vi "ZK仪器状态.vi"(7 "运行模式":string, 8 "error in (no error)":errorcluster, 11 "Slave ID":T3) -> (0 "error out":errorcluster, 2 "质控仪器状态显示":T1, 3 "质控仪器状态":T2 {"当前步骤数" format="0x%04xH"})   [LabVIEW 2016, in "质控单元V4.lvlib"]
uses:
  <vilib>/Plasmionique/MB Master/MB_Master/MB_Master.lvclass
  <vilib>/Plasmionique/MB Master/MB Master.lvlib
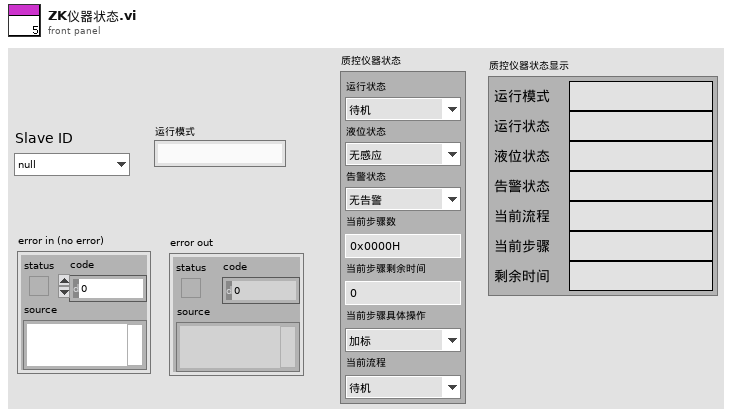
[diagram p1: front panel]
types:
  T1 = typedef "质控单元V4.lvlib/质控仪器状态显示.ctl" = cluster{"运行模式":string, "运行状态":string, "液位状态":string, "告警状态":string, "当前流程":string, "当前步骤":string, "剩余时间":string}
  T2 = typedef "质控单元V4.lvlib/质控仪器状态.ctl" = cluster{"运行状态":enum16{"待机", "润洗", "进样", "定量", "加标", "等待取样", "排液", "异常停机"}, "液位状态":enum16{"无感应", "有感应"}, "告警状态":enum16{"无告警", "液位故障告警", "注射泵异常"}, "当前步骤数":u16, "当前步骤剩余时间":u16, "当前步骤具体操作":enum16{"加标", "进样", "排液", "搅拌", "定量"}, "当前流程":enum16{"待机", "进样流程", "加标流程", "排液流程", "水样润洗流程", "加标润洗流程"}}
  T3 = typedef "质控单元V4.lvlib/质控slave id.ctl" = enum16{"null", "氨氮", "总磷", "总氮", "CODMn", "CODCr"}
  T4 = cluster{"[0]":u16, "[1]":u16, "[2]":u16, "[3]":u16, "[4]":u16, "[5]":u16, "[6]":u16}
  T5 = enum16{"待机", "润洗", "进样", "定量", "加标", "等待取样", "排液", "异常停机"}
  T6 = cluster{"运行模式":string, "RingText.Text":string, "RingText.Text":string, "RingText.Text":string, string, "RingText.Text":string, string}
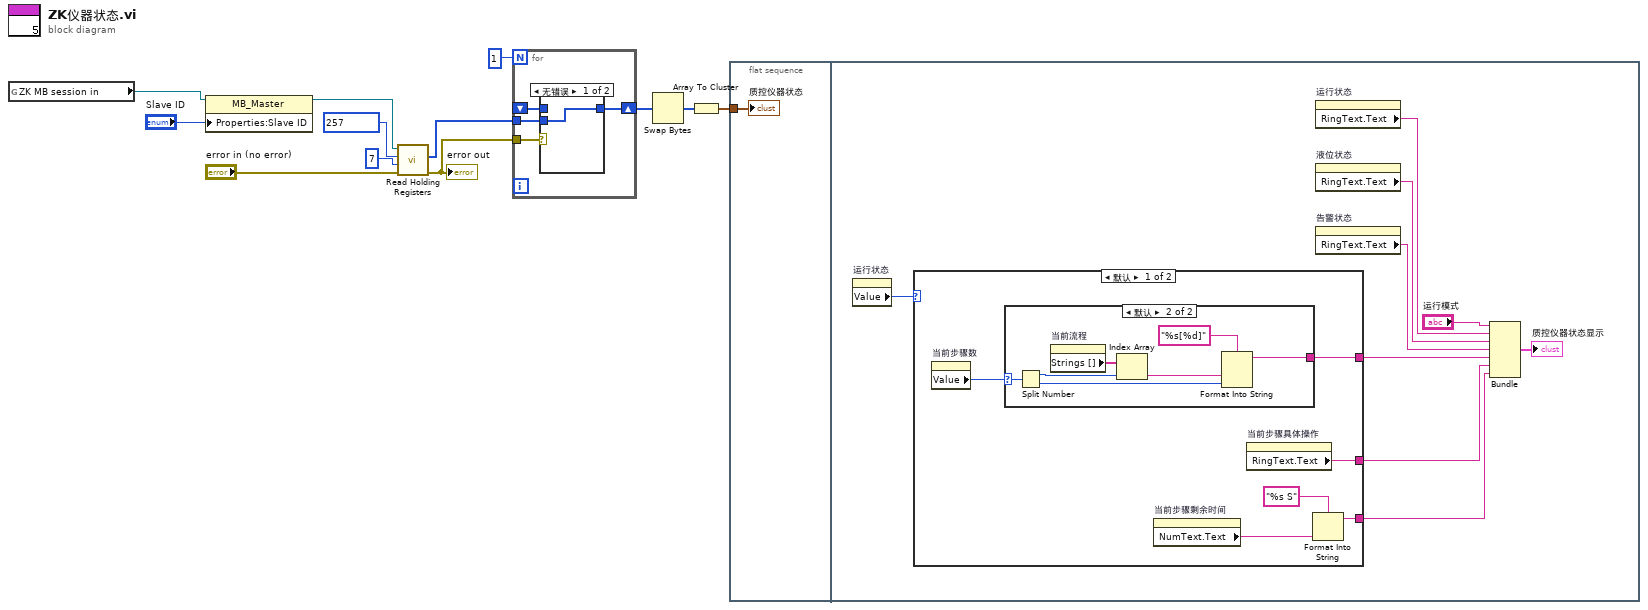
[diagram p0: block diagram]
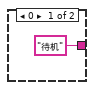
[diagram p2: hidden frame]
diagram:
  n1 = global read "ZK非断电保存全局变量.vi" "ZK MB session in"() -> (w11:refnum<class "MB_Master.lvclass">)
  n2 = property class="MB_Master"(reference=w11, "Properties:Slave ID"="Slave ID") -> (reference out=w9:refnum<class "MB_Master.lvclass">)  [unwired: 1 in, 1 out]
  n3 = call <vilib>:"Read Holding Registers.vi"("error in (no error)"="error in (no error)", "quantity"=u16 7, "starting address"=u16 257, "MB session in"=w9) -> ("error out"=w6:errorcluster, "Registers"=w5:u16[])  [unwired: 5 in, 1 out]
  "error out" <- w6
  n4 = for {
    N: 1 -> [_]
    tunnel: w6 -> [w16]
    tunnel: w5 -> [w15]
    shift-right: [w14] -> w4
    shift-left: _ -> [w13]
    n5 = case shown="无错误" w16 {
      tunnel: w15 -> [w17 _]
      tunnel: [w17 w18] -> w14
      tunnel: w13 -> [_ w18]
      frame No Error {
      }
      frame Error {
      }
    }
  }
  n6 = Swap Bytes(anything=w4) -> (byte swapped=w3:u16[])
  n7 = Array To Cluster(array=w3) -> (cluster=w2:T4)
  n8 = flat-sequence {
    tunnel: w2 -> [w19]
    frame #0 {
      "质控仪器状态" <- w19
    }
    frame #1 {
      n9 = property on="运行状态" class="Enum (严格)"() -> ("Value"=w21:T5)  [unwired: 2 in, 2 out]
      n10 = case shown="默认" w21 {
        tunnel: [w34 _] -> w25
        tunnel: [w33 _] -> w24
        tunnel: [w30 _] -> w23
        frame Default {
          n11 = property on="当前步骤数" class="DigNum (严格)"() -> ("Value"=w29:u16)  [unwired: 2 in, 2 out]
          n12 = case shown="默认" w29 {
            selector: w29 -> [_ w36]
            tunnel: ["待机" w37] -> w34
            frame 0 {
            }
            frame Default {
              n13 = Split Number(x=w36) -> (hi(x)=w41:u8, lo(x)=w39:u8)
              n14 = property on="当前流程" class="Enum (严格)"() -> ("Strings []"=w40:string[])  [unwired: 2 in, 2 out]
              n15 = Index Array(array=w40, index=w41) -> (element=w42:string)
              n16 = Format Into String(format string="%s[%d]" ("格式字符串"), w42, w39) -> (resulting string=w37:string)  [unwired: 2 in, 1 out]
            }
          }
          n17 = property on="当前步骤剩余时间" class="DigNum (严格)"() -> ("NumText.Text"=w31:string)  [unwired: 2 in, 2 out]
          n18 = property on="当前步骤具体操作" class="Enum (严格)"() -> ("RingText.Text"=w33:string)  [unwired: 2 in, 2 out]
          n19 = Format Into String(format string="%s S" ("格式字符串"), w31) -> (resulting string=w30:string)  [unwired: 2 in, 1 out]
        }
        frame "待机", "等待取样" {
        }
      }
      n20 = property on="运行状态" class="Enum (严格)"() -> ("RingText.Text"=w28:string)  [unwired: 2 in, 2 out]
      n21 = property on="液位状态" class="Enum (严格)"() -> ("RingText.Text"=w27:string)  [unwired: 2 in, 2 out]
      n22 = property on="告警状态" class="Enum (严格)"() -> ("RingText.Text"=w26:string)  [unwired: 2 in, 2 out]
      n23 = Bundle("运行模式"="运行模式", "RingText.Text"=w28, "RingText.Text"=w27, "RingText.Text"=w26, w25, "RingText.Text"=w24, w23) -> (→"质控仪器状态显示":T6)  [unwired: 1 in]
    }
  }
